vi "XML_slow.vi"(1 "Slow Cluster":T1={"Number of Slow Parameters"=0, "UTC format?"=TRUE, "Sensor Upper bounds"=[85, 1000000, 8000, 8000, 8000, 14000, 99, 33000], "Sensor Lower bounds"=[-40, 0, -8000, -8000, -8000, -14000, 0, -33000], "datanames"=[], "Descriptions"=[]}, 2 "Input String":string) -> (0 "Output String":string)   [LabVIEW 2012]
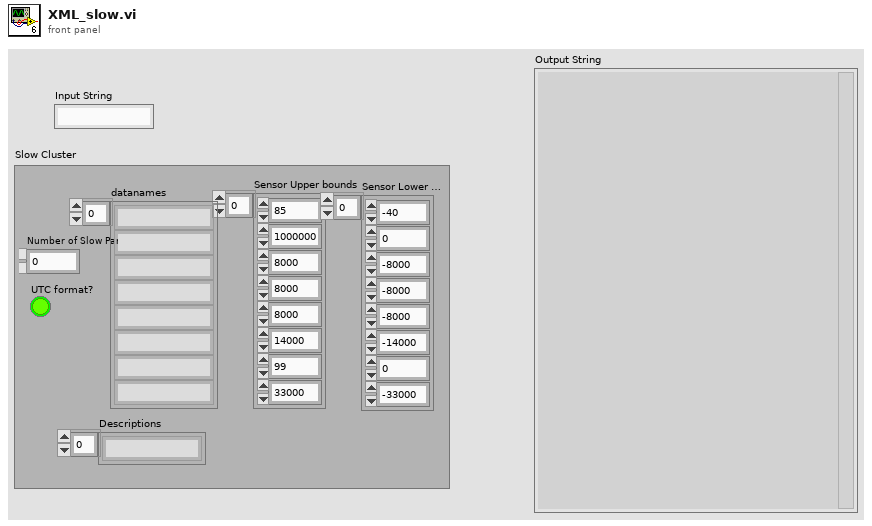
[diagram p1: front panel]
types:
  T1 = cluster{"Number of Slow Parameters":i32, "UTC format?":bool, "Sensor Upper bounds":i32[], "Sensor Lower bounds":i32[], "datanames":string[], "Descriptions":string[]}
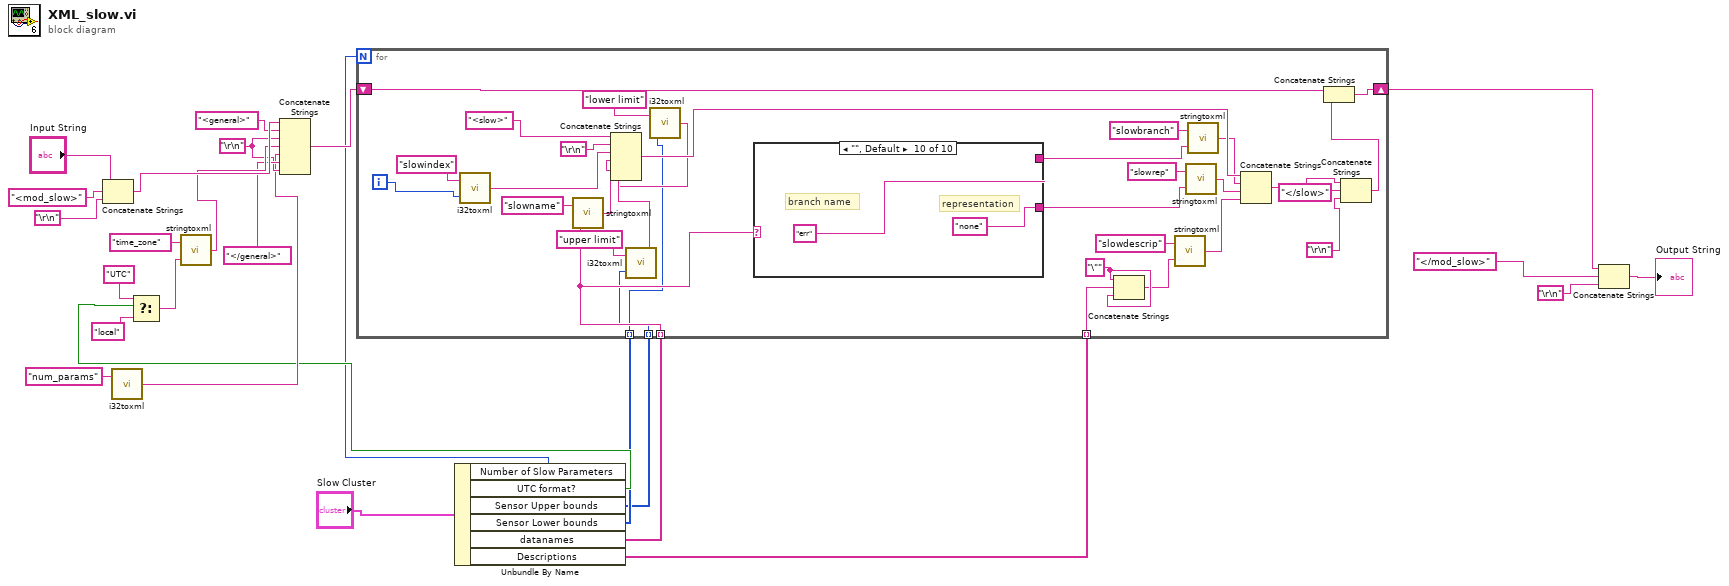
[diagram p0: block diagram]
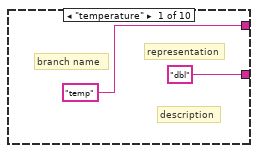
[diagram p2: hidden frame]
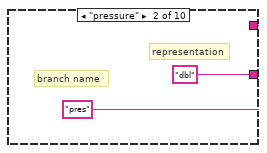
[diagram p3: hidden frame]
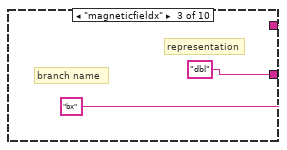
[diagram p4: hidden frame]
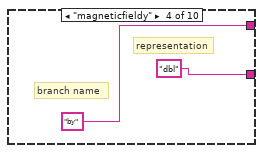
[diagram p5: hidden frame]
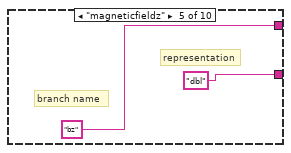
[diagram p6: hidden frame]
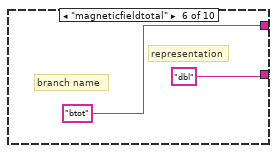
[diagram p7: hidden frame]
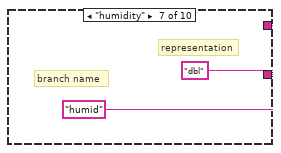
[diagram p8: hidden frame]
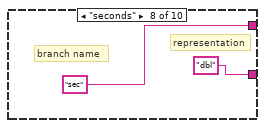
[diagram p9: hidden frame]
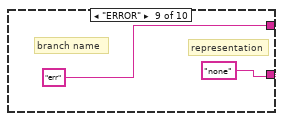
[diagram p10: hidden frame]
diagram:
  w16 = "\r\n"
  n1 = Concatenate Strings("Input String", "<mod_slow>", "\r\n") -> (w20:string)
  n2 = call "i32toxml.vi"("variable name"="num_params") -> ("xml string"=w12:string)  [unwired: 1 in]
  n3 = Unbundle By Name("Slow Cluster") -> ("Number of Slow Parameters"=w6:i32, "UTC format?"=w7:bool, "Sensor Upper bounds"=w4:i32[], "Sensor Lower bounds"=w5:i32[], "datanames"=w3:string[], "Descriptions"=w1:string[])
  n4 = Select(t="UTC" ("XML Tag"), s=w7, f="local") -> (s? t:f=w25:string)
  n5 = call "stringtoxml.vi"("String to write"=w25, "XML Tag"="time_zone") -> ("xml string"=w18:string)
  n6 = Concatenate Strings(w20, "<general>", w16, w18, w12, "</general>" ("string"), w16) -> (w11:string)
  n7 = for {
    N: w6 -> [_]
    shift-right: [w49] -> w9
    shift-left: w11 -> [w58]
    tunnel: w5 -> [w29] mode=indexing
    tunnel: w4 -> [w28] mode=indexing
    tunnel: w3 -> [w30] mode=indexing
    tunnel: w1 -> [w27] mode=indexing
    i -> [w31]
    w46 = "\"" ("string")
    n8 = call "i32toxml.vi"("variable"=w31, "variable name"="slowindex") -> ("xml string"=w37:string)
    n9 = call "stringtoxml.vi"("String to write"=w30, "XML Tag"="slowname") -> ("xml string"=w48:string)
    n10 = call "i32toxml.vi"("variable"=w28, "variable name"="upper limit") -> ("xml string"=w34:string)
    n11 = call "i32toxml.vi"("variable"=w29, "variable name"="lower limit") -> ("xml string"=w32:string)
    n12 = Concatenate Strings("<slow>" ("string"), "\r\n", w37, w48, w34, w32) -> (w44:string)
    n13 = case shown="\"\", Default" w30 {
      tunnel: ["dbl" ("XML Tag") "dbl" ("XML Tag") "dbl" ("XML Tag") "dbl" ("XML Tag") "dbl" ("XML Tag") "dbl" ("XML Tag") "dbl" ("XML Tag") "dbl" ("XML Tag") "none" ("XML Tag") "none" ("XML Tag")] -> w54
      tunnel: ["temp" "pres" "bx" "by" "bz" "btot" "humid" "sec" "err" "err"] -> w41
      frame "temperature" {
        # "branch name"
        # "description"
        # "representation"
      }
      frame "pressure" {
        # "branch name"
        # "representation"
      }
      frame "magneticfieldx" {
        # "branch name"
        # "representation"
      }
      frame "magneticfieldy" {
        # "branch name"
        # "representation"
      }
      frame "magneticfieldz" {
        # "branch name"
        # "representation"
      }
      frame "magneticfieldtotal" {
        # "branch name"
        # "representation"
      }
      frame "humidity" {
        # "branch name"
        # "representation"
      }
      frame "seconds" {
        # "branch name"
        # "representation"
      }
      frame "ERROR" {
        # "branch name"
        # "representation"
      }
      frame "", Default {
        # "branch name"
        # "representation"
      }
    }
    n14 = Concatenate Strings(w46, w27, w46) -> (w45:string)
    n15 = call "stringtoxml.vi"("String to write"=w45, "XML Tag"="slowdescrip") -> ("xml string"=w52:string)
    n16 = call "stringtoxml.vi"("String to write"=w54, "XML Tag"="slowrep") -> ("xml string"=w53:string)
    n17 = call "stringtoxml.vi"("String to write"=w41, "XML Tag"="slowbranch") -> ("xml string"=w43:string)
    n18 = Concatenate Strings(w44, w43, w53, w52) -> (w47:string)
    n19 = Concatenate Strings(w47, "</slow>" ("string"), "\r\n") -> (w50:string)
    n20 = Concatenate Strings(w58, w50) -> (w49:string)
  }
  n21 = Concatenate Strings(w9, "</mod_slow>" ("string"), "\r\n") -> (→"Output String":string)
